vi "SQL Query.vi"(8 "error in (no error)":errorcluster, 10 "SQL Query":string, 11 "ADODB in":refnum<class "ADODB.lvclass">) -> (0 "error out":errorcluster, 2 "Query Result":string[][](array[string]), 3 "ADODB out":refnum<class "ADODB.lvclass">)   [LabVIEW 2020, in "ADODB.lvlib" / "ADODB.lvclass"]
uses:
  ADODB.lvclass
  ADODB.lvclass/ADODB.ctl
  <vilib>/addons/database/Connection.llb/Conn Execute.vi
  <vilib>/addons/database/Recordset.llb/Rec Fetch Recordset Data (R).vi
  <vilib>/addons/database/Recordset.llb/Rec Destroy - Connection.vi
  <vilib>/addons/database/_DB Variant To Data/Database Variant To Data.xnode
  <vilib>/addons/database/NI_Database_API.lvlib
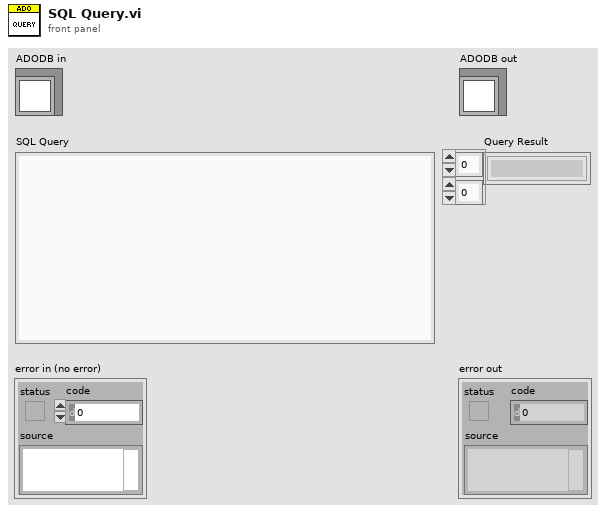
[diagram p1: front panel]
types:
  T1 = typedef "NI_Database_API.lvlib/Conn ObjectReference.ctl" = refnum<k1>
  T2 = typedef "NI_Database_API.lvlib/Rec ObjectReference.ctl" = refnum<k1>
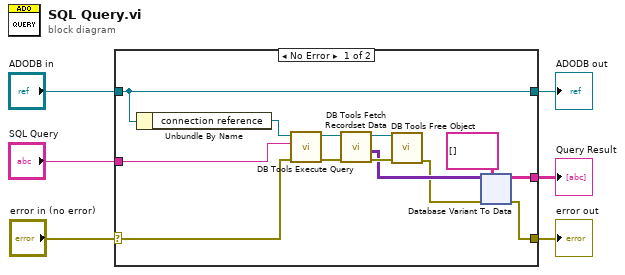
[diagram p0: block diagram]
diagram:
  n1 = case shown="No Error" "error in (no error)" {
    selector: "error in (no error)" -> [w11 w65]
    tunnel: [w8 w65] -> w5
    tunnel: "ADODB in" -> [w10 w64]
    tunnel: [w10 w64] -> w3
    tunnel: "SQL Query" -> [w7 _]
    tunnel: [w12 _] -> w1
    frame No Error {
      n2 = Unbundle By Name(w10) -> ("connection reference"=w19:T1)
      n3 = call-poly <vilib>:"DB Tools Execute Query.vi"("error in (no error)"=w11, "SQL query"=w7, "connection reference"=w19) -> ("error out"=w18:errorcluster, "recordset reference"=w17:T2)  [unwired: 5 in]
      n4 = call-poly <vilib>:"DB Tools Fetch Recordset Data.vi"("error in (no error)"=w18, "recordset reference"=w17) -> ("error out"=w16:errorcluster, "recordset data"=w13:variant[][], "recordset reference out"=w15:T2)  [unwired: 3 in]
      n5 = call-poly <vilib>:"DB Tools Free Object.vi"("error in (no error)"=w16, "recordset reference"=w15) -> ("error out"=w9:errorcluster)  [unwired: 8 in, 1 out]
      n6 = xnode "Database Variant To Data"("database variant"=w13, "error in (no error)"=w9, "type"=string[][] [] ("Query Result")) -> ("data"=w12:string[][], "error out"=w8:errorcluster)
    }
    frame Error {
    }
  }
  "error out" <- w5
  "ADODB out" <- w3
  "Query Result" <- w1
